vi "Module Type.vi"(11 "EStop Module in":refnum<class "EStop Module.lvclass">) -> (2 "Module Type":string)   [LabVIEW 2020, in "VolatusControl.lvlib" / "EStop Module.lvclass"]
uses:
  EStop Module.lvclass
  EStop Module.lvclass/EStop Module.ctl
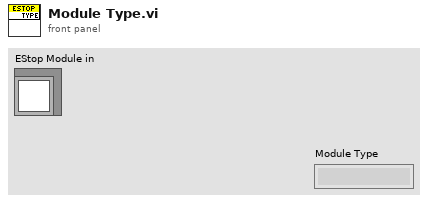
[diagram p1: front panel]
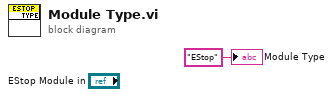
[diagram p0: block diagram]
diagram:
  "Module Type" <- "EStop" ("Module Type")
